vi "VM Monitor.vi"() -> ()   [LabVIEW 2022 SP3]
uses:
  <vilib>/Utility/sysdir.llb/System Directory Type.ctl
  <instrlib>/tio-labview/TIO Library/TIO Stream Open.vi
  <instrlib>/tio-labview/TIO Library/TIO RPC Send REQuest.vi
  <instrlib>/tio-labview/Labview Signal Processing/Log Binning.vi
  <instrlib>/tio-labview/TIO Library/TIO RPC Notification.vi
  <vilib>/Utility/error.llb/Clear Errors.vi
  <instrlib>/tio-labview/TIO Library/TIO RPC Parse Reply.vi
  <instrlib>/tio-labview/TIO Library/TIO RPC Parse Reply Error.vi
  <instrlib>/tio-labview/TIO Library/TIO Data Stream Parse timebase Info.vi
  <instrlib>/tio-labview/TIO Library/TIO Data Stream Parse pstream Info.vi
  <instrlib>/tio-labview/TIO Library/TIO Data Stream Parse dstream Info.vi
  <vilib>/Utility/High Resolution Relative Seconds.vi
  <instrlib>/tio-labview/TIO Library/TIO Serial Port Name Search.vi
  <instrlib>/tio-labview/TIO Library/TIO Stream Write.vi
  <instrlib>/tio-labview/TIO Library/TIO RPC Form Request.vi
  <instrlib>/tio-labview/Labview Signal Processing/Log Range.vi
  <instrlib>/tio-labview/TIO Library/TIO SLIP Serial Write.vi
  <instrlib>/tio-labview/TIO Library/TIO Form Packet.vi
  <instrlib>/tio-labview/TIO Library/TIO SLIP Encode.vi
  <instrlib>/tio-labview/TIO Library/TIO Serial Checksum CRC32.vi
  <vilib>/Utility/tcp.llb/UDP Multicast Open.vi
  <vilib>/Utility/tcp.llb/UDP Multicast Read-Write Open.vi
  <instrlib>/tio-labview/TIO Library/TIO Serial Port Discovery.vi
  <vilib>/Instr/_visa.llb/VISA Configure Serial Port (Instr).vi
  <instrlib>/tio-labview/TIO Library/TIO RPC Blocking.vi
  <vilib>/Analysis/6fits.llb/General Polynomial Fit.vi
  <vilib>/measure/maspectr.llb/FFT Power Spectrum and PSD.vi
  <vilib>/measure/maspectr.llb/FFT Power Spectrum and PSD for 1 Chan.vi
  <instrlib>/tio-labview/TIO Library/TIO Stream Read Non-blocking.vi
  <instrlib>/tio-labview/TIO Library/TIO RPC Send Heartbeat.vi
panel:
  in  "Data Rate":dbl[unit]=1000.0
  in  "Reset":bool
  in  "Log":bool
  in  "Log to file":path
  in  "URL":refnum<visa-resource-name>="tcp://localhost"
  in  "Quit":bool
  in  "Duration":dbl[unit]=1000.0
  out "T":dbl[unit]=35.88999938964844 format="%_4g"
  out "gz":dbl[unit]=-0.004659709835278764 format="%_4p"
  out "gy":dbl[unit]=-0.022590839449213182 format="%_4p"
  out "gx":dbl[unit]=-0.019901542485926807 format="%_4p"
  out "az":dbl[unit]=0.00052925927734375 format="%_4g"
  out "ay":dbl[unit]=-0.00082588623046875 format="%_4g"
  out "ax":dbl[unit]=9.998315429687501e-05 format="%_4g"
  out "P":dbl[unit]=106140.01245117188 format="%_6g"
  out "BX":dbl[unit]=3.6740006401538853e-09 format="%_6g"
  out "BY":dbl[unit]=-5.247936037597656e-07 format="%_6g"
  out "BZ":dbl[unit]=-4.973549954223633e-07 format="%_6g"
  out "B":dbl[unit]=7.230379266504588e-07 format="%_6g"
  out "Field X":T1(graph)
  out "Field Y":T1(graph)
  out "Field Z":T1(graph)
  out "Field Total":T1(graph)
  out "ID":string="Twinleaf VM4 R4"
  in  "Bin":bool=TRUE
  out "XY Graph":T2(graph)
  # "VM Monitor"
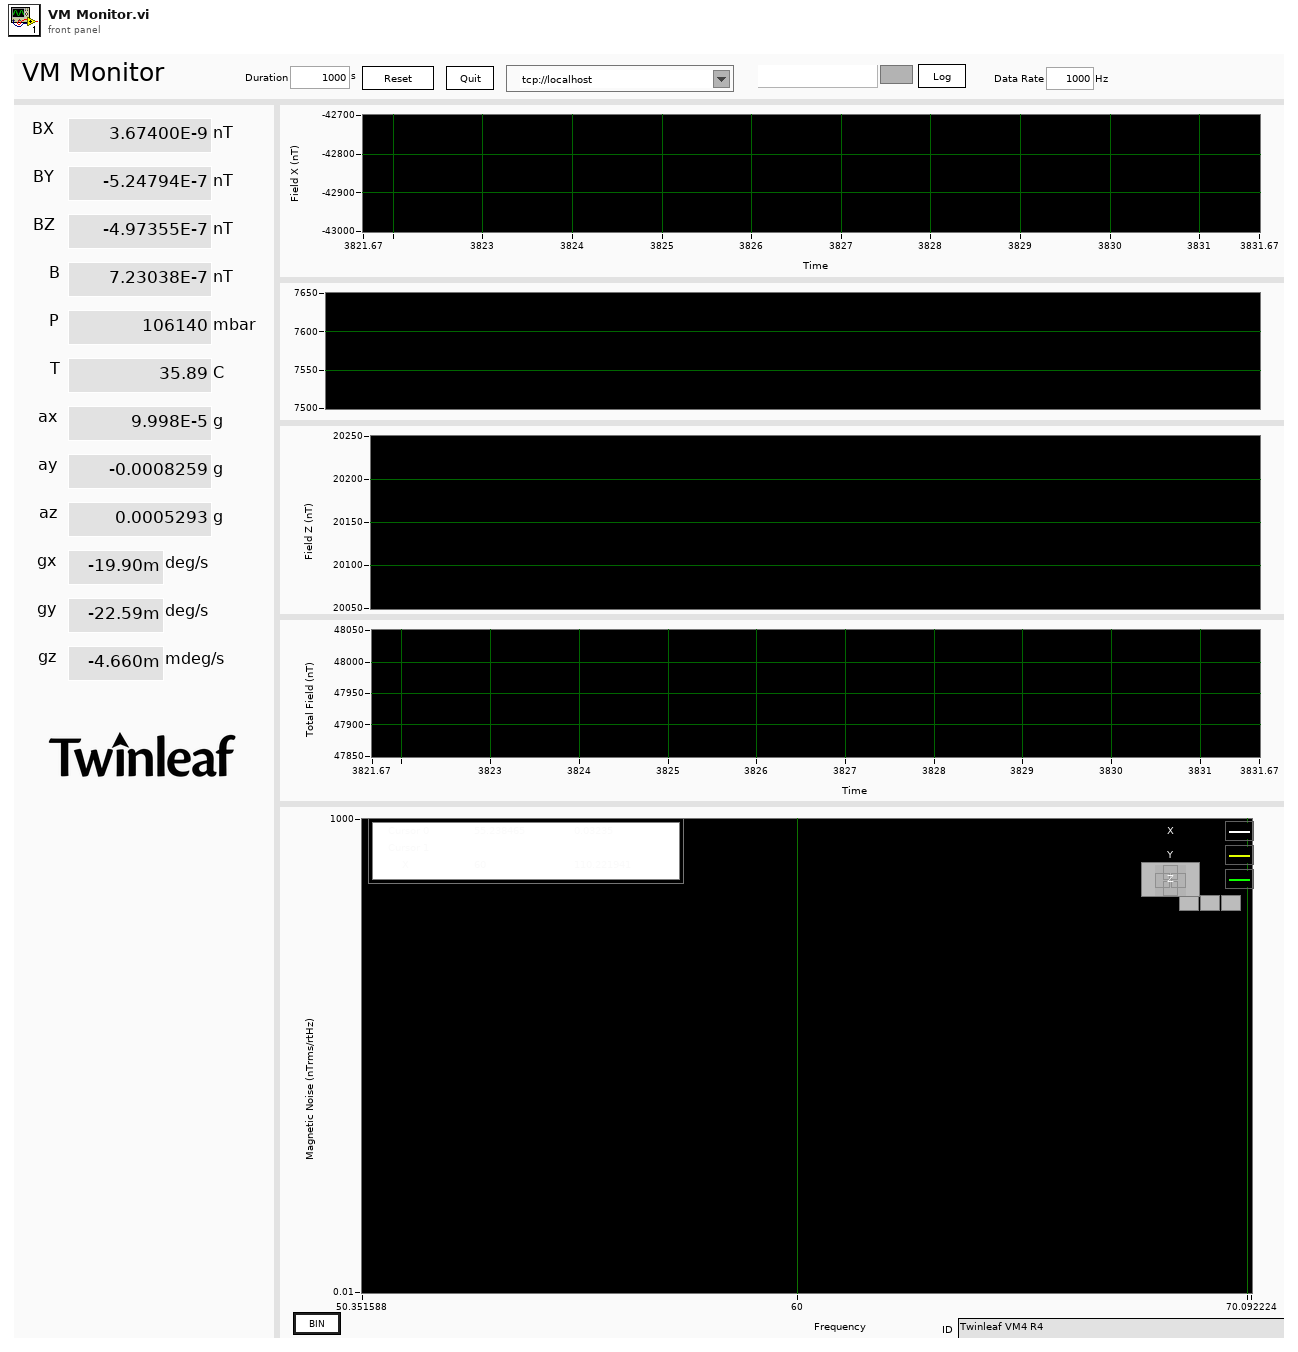
[diagram p1: front panel]
types:
  T1 = cluster{"start":dbl, "dt":dbl, "Timeseries":dbl[]}
  T2 = cluster{"Frequencies Binned":dbl[], "Spectrum Binned":dbl[]}[]
  T3 = cluster{"Awaiting REP":bool, "REQ ID":u32, "streams in":cluster{"id":u16, "timebase id":u16, "period":u32, "offset":u32, "sample number":u64, "total components":u16, "flags":u16, "components":cluster{"source id":u16, "flags":u16, "period":u32, "offset":u32}[]}[], "sources":cluster{"id":u16, "timebase_id":u16, "period":u32, "offset":u32, "fmt":i32, "flags":u16, "channels":u16, "type":u8, "name":string, "column names":string[], "title":string, "units":string}[], "timebases":cluster{"id":u16, "source":u8, "epoch":u8, "start time":u64, "period numerator (µs)":u32, "period denominator (µs)":u32, "flags":u32, "stability":sgl, "source id":string}[]}
  T4 = typedef "System Directory Type.ctl" = i32
  T5 = cluster{"TS Connection":cluster{"Type":enum16{"Serial", "TCP", "UDP", "mUDP"}, "URL":refnum<visa-resource-name>, "TO":u32, "Addr":u32, "Port":i32, "TCP":refnum<k5>, "UDP":refnum<k16>, "Route":string}, "REQ":refnum<queue>, "REP":refnum<queue>}
  T6 = cluster{"start":dbl, "dt":dbl, "Timeseries":sgl[][]}
  T7 = cluster{"stream ID":u16, "Sample Number":u32, "Raw Data":string}
  T8 = cluster{"TC Connection":cluster{"Type":enum16{"Serial", "TCP", "UDP", "mUDP"}, "URL":refnum<visa-resource-name>, "TO":u32, "Addr":u32, "Port":i32, "TCP":refnum<k5>, "UDP":refnum<k16>, "Route":string}, "REQ":refnum<queue>, "REP":refnum<queue>}
  T9 = cluster{"Name":string, "Waveform":cluster{"start":dbl, "dt":dbl, "Timeseries":dbl[][]}}[]
  T10 = cluster{"start":dbl, "dt":dbl, "Timeseries":dbl[][]}
  T11 = cluster{"Frequencies Binned":dbl[], "Spectrum Binned":dbl[]}
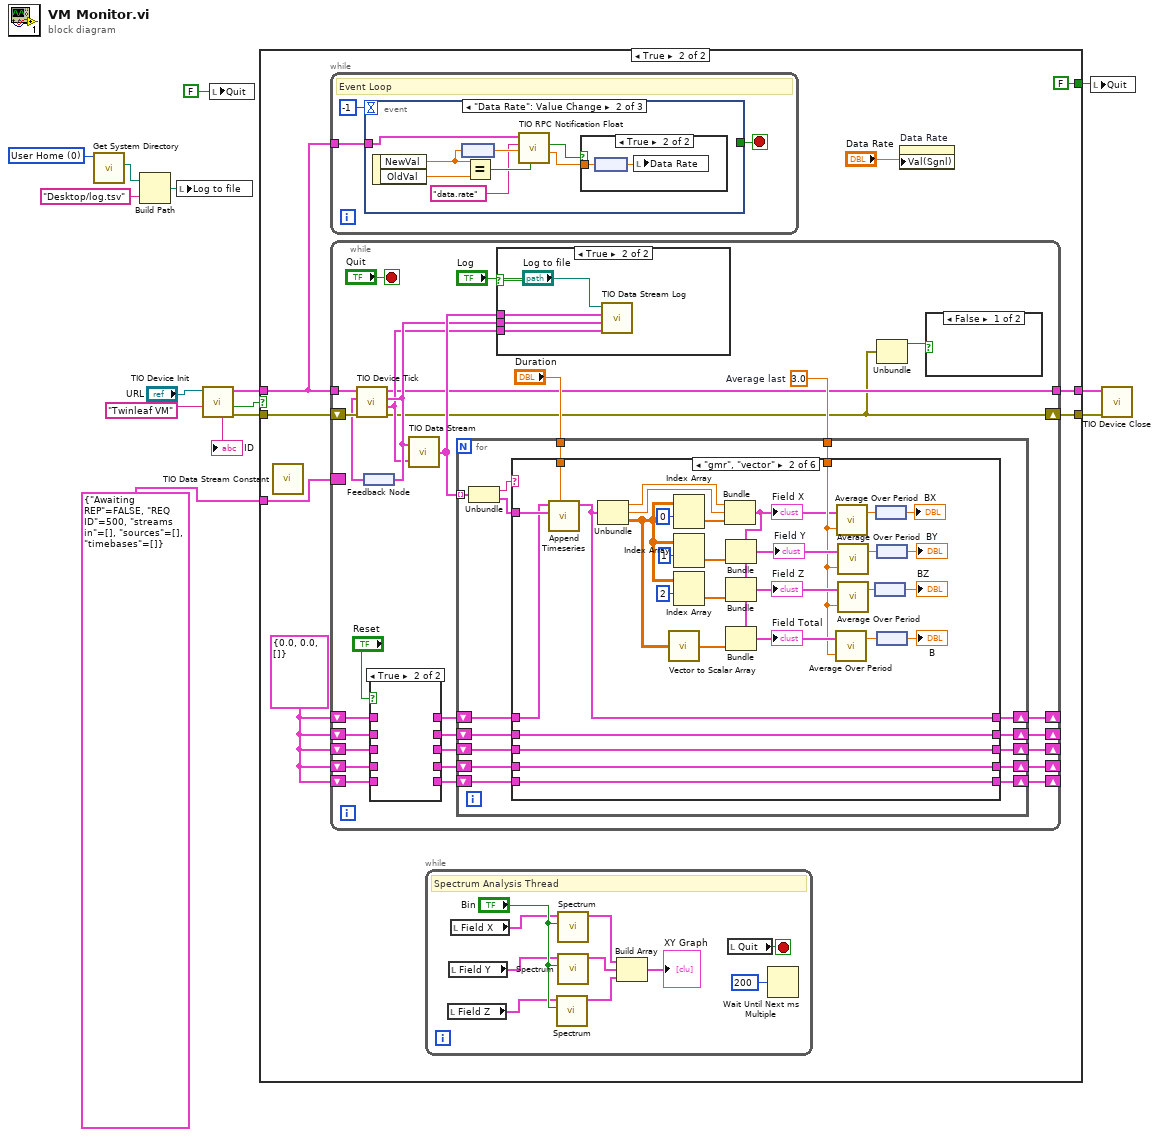
[diagram p0: block diagram]
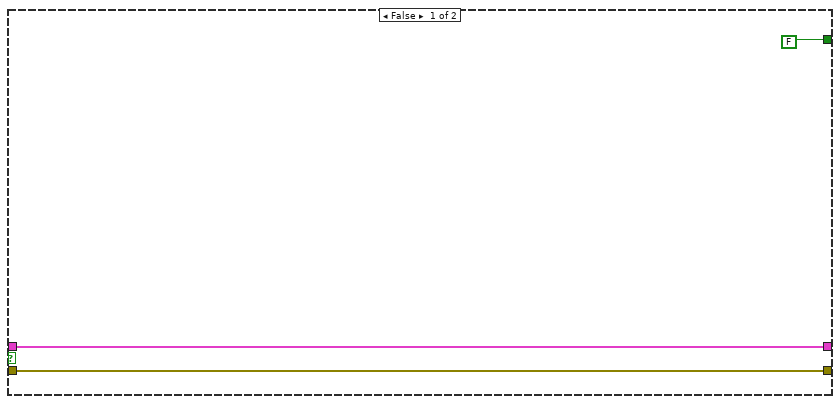
[diagram p2: hidden frame]
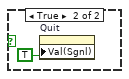
[diagram p3: hidden frame]
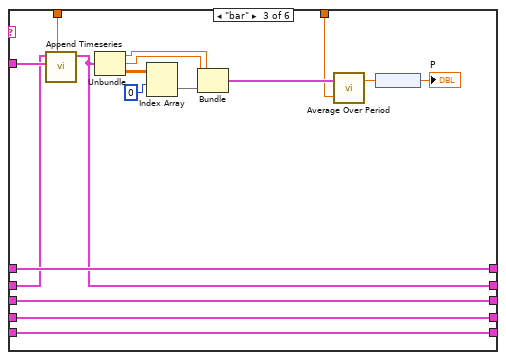
[diagram p6: hidden frame]
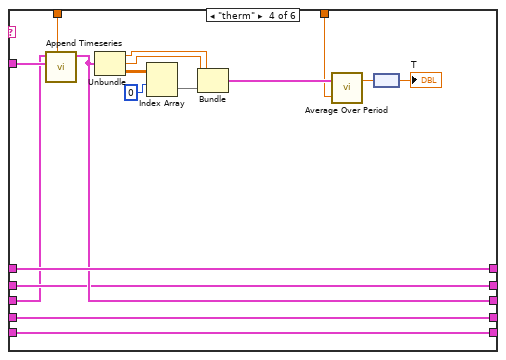
[diagram p7: hidden frame]
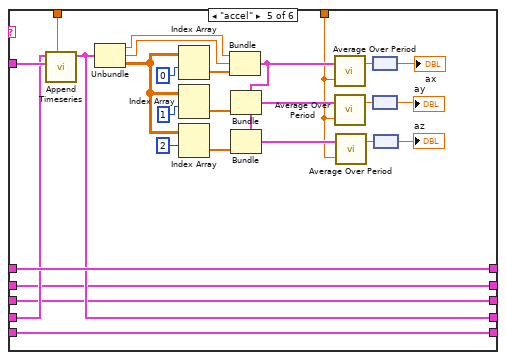
[diagram p8: hidden frame]
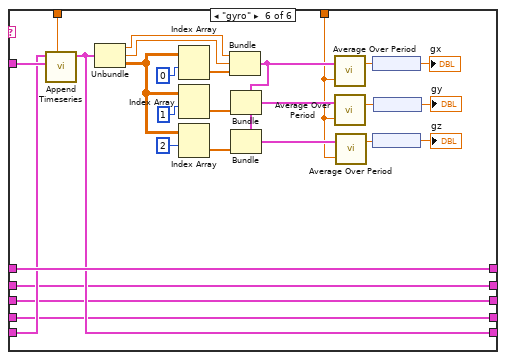
[diagram p9: hidden frame]
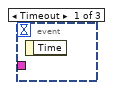
[diagram p11: hidden frame]
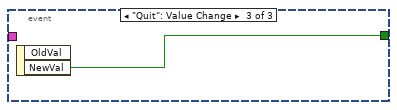
[diagram p13: hidden frame]
diagram:
  w9 = T4 0 items=["User Home"=0, "User Desktop"=1, "User Documents"=2, "User Application Data"=3, "User Preferences"=4, "User Temporary"=5, "Public Documents"=6, "Public Application Data"=7, "Public Preferences"=8, "Public Cache"=13, "System Core Libraries"=9, "System Installed Libraries"=10, "Application Files"=11, "Boot Volume Root"=12] ("system directory type")
  n1 = call <vilib>:"Get System Directory.vi"("system directory type"=w9) -> ("system directory"=w8:path)  [unwired: 10 in]
  n2 = Build Path(base path=w8, name or relative path="Desktop/log.tsv") -> (appended path=w6:path)
  n3 = local write "Log to file"(w6) -> ()
  n4 = call <instrlib>:"TIO Device Init.vi"("ID"="Twinleaf VM" ("Prefix"), "URL"="URL") -> ("error out"=w14:errorcluster, "Connected"=w2:bool, "TIO"=w15:T5, "ID Verified"=→"ID":string)  [unwired: 5 in, 1 out]
  n5 = local write "Quit"(FALSE ("Kill")) -> ()
  n6 = case shown="True" w2 {
    tunnel: w15 -> [w17 w25]
    tunnel: w14 -> [w16 w26]
    tunnel: [FALSE FALSE ("Kill")] -> w10
    tunnel: [w17 w22] -> w4
    tunnel: [w16 w21] -> w5
    tunnel: T3 {"Awaiting REP"=FALSE, "REQ ID"=500, "streams in"=[], "sources"=[], "timebases"=[]} ("TIO State") -> [_ w20]
    frame False {
    }
    frame True {
      w23 = T6 {"start"=0.0, "dt"=0.0, "Timeseries"=[]}
      n7 = call <instrlib>:"TIO Data Stream Constant.vi"() -> ()  [unwired: 1 out]
      n8 = while {
        tunnel: w25 -> [w206]
        stop <- w205 stop-if-true
        # "Event Loop"
        n9 = event shown="[1] \"Data Rate\": Value Change" {
          selector: _ -> [_ _ _]
          dyn-events: _ -> [_ _ _]
          timeout: -1 -> [_ _ _]
          tunnel: w206 -> [_ w210 _]
          tunnel: [_ _ w218] -> w205
          event Timeout {
            n10 = event-data() -> ()  [unwired: 1 in, 1 out]
          }
          event "Data Rate": Value Change {
            n11 = event-data() -> ("NewVal"=w212:dbl[unit], "OldVal"=w214:dbl[unit])  [unwired: 1 in]
            n12 = node(w212) -> (w211:dbl)
            n13 = Equal?(x=w212, y=w214) -> (x = y?=w215:bool)
            n14 = call <instrlib>:"TIO RPC Notification Float.vi"("Read"=w215, "Set value"=w211, "Topic"="data.rate", "TIO"=w210) -> ("Get value (default if error)"=w213:sgl, "Response"=w208:bool)  [unwired: 4 in, 1 out]
            n15 = case shown="True" w208 {
              tunnel: w213 -> [_ w217]
              frame False {
              }
              frame True {
                n16 = node(w217) -> (w216:sgl[unit])
                n17 = local write "Data Rate"(w216) -> ()
              }
            }
          }
          event "Quit": Value Change {
            n18 = event-data() -> ("NewVal"=w218:bool)  [unwired: 1 in, 1 out]
          }
        }
      }
      n19 = while {
        tunnel: w25 -> [w55]
        shift-right: [w51] -> _
        shift-left: w23 -> [w39]
        shift-right: [w48] -> _
        shift-left: w23 -> [w38]
        shift-right: [w47] -> _
        shift-left: w23 -> [w37]
        shift-right: [w46] -> _
        shift-left: w23 -> [w36]
        shift-right: [w45] -> _
        shift-left: w23 -> [w35]
        border: w20 -> [_]
        tunnel: [w29] -> w22
        shift-right: [w28] -> w21
        shift-left: w26 -> [w54]
        stop <- "Quit" stop-if-true
        w50 = dbl[unit] 3.0  # Average last
        n20 = feedback #1() -> (w44:T3)
        n21 = call <instrlib>:"TIO Device Tick.vi"("Error in"=w54, "TIO State"=w44, "TIO"=w55) -> ("Error out"=w28:errorcluster, "Data Out"=w41:T7, "TIO State"=w42:T3, "TIO"=w29:T8)  [unwired: 5 in]
        n22 = feedback-in #1(w42) -> ()
        n23 = case shown="True" "Reset" {
          tunnel: w39 -> [w61 _]
          tunnel: w38 -> [w60 _]
          tunnel: w37 -> [w59 _]
          tunnel: w36 -> [w58 _]
          tunnel: w35 -> [w57 _]
          tunnel: [w57 _] -> w34
          tunnel: [w58 _] -> w33
          tunnel: [w59 _] -> w32
          tunnel: [w60 _] -> w31
          tunnel: [w61 _] -> w30
          frame False {
          }
          frame True {
          }
        }
        n24 = call <instrlib>:"TIO Data Stream.vi"("Raw Data"=w41, "TIO State"=w42) -> ("Data Out"=w43:T9)
        n25 = for {
          tunnel: "Duration" -> [w76]
          tunnel: w50 -> [w73]
          tunnel: w43 -> [w64] mode=indexing
          shift-right: [w75] -> w51
          shift-left: w30 -> [w74]
          shift-right: [w72] -> w48
          shift-left: w31 -> [w71]
          shift-right: [w70] -> w47
          shift-left: w32 -> [w69]
          shift-right: [w68] -> w46
          shift-left: w33 -> [w67]
          shift-right: [w66] -> w45
          shift-left: w34 -> [w65]
          n26 = Unbundle(w64) -> ("Name"=w63:string, "Waveform"=w62:T10)
          n27 = case shown="\"gmr\", \"vector\"" w63 {
            tunnel: w76 -> [_ w112 w129 w146 w173 w200]
            tunnel: w73 -> [_ w93 w118 w136 w152 w185]
            tunnel: w62 -> [_ w88 w122 w140 w156 w189]
            tunnel: [w81 w87 w121 w139 w153 w186] -> w75
            tunnel: w74 -> [w81 w86 w121 w139 w153 w186]
            tunnel: [w80 w85 w117 w133 w149 w176] -> w72
            tunnel: w71 -> [w80 w85 w116 w133 w149 w176]
            tunnel: [w79 w84 w115 w134 w148 w175] -> w70
            tunnel: w69 -> [w79 w84 w115 w132 w148 w175]
            tunnel: [w78 w83 w114 w131 w151 w174] -> w68
            tunnel: w67 -> [w78 w83 w114 w131 w150 w174]
            tunnel: [w77 w82 w113 w130 w147 w178] -> w66
            tunnel: w65 -> [w77 w82 w113 w130 w147 w177]
            frame Default {
            }
            frame "gmr", "vector" {
              n28 = call <instrlib>:"Append Timeseries.vi"("Duration"=w112, "In New"=w88, "In Old"=w86) -> ("Appended"=w87:T10)  [unwired: 8 in]
              n29 = Unbundle(w87) -> ("start"=w111:dbl, "dt"=w92:dbl, "Timeseries"=w90:dbl[][])
              n30 = call <instrlib>:"Vector to Scalar Array.vi"("Three axis vector"=w90) -> ("Total field"=w89:dbl[])
              n31 = Index Array(array=w90, index (row)=0 ("disabled index (col)")) -> (element=w107:dbl[])  [unwired: 1 in]
              n32 = Index Array(array=w90, index (row)=1 ("disabled index (col)")) -> (element=w106:dbl[])  [unwired: 1 in]
              n33 = Index Array(array=w90, index (row)=2 ("disabled index (col)")) -> (element=w105:dbl[])  [unwired: 1 in]
              n34 = Bundle("start"=w111, "dt"=w92, "Timeseries"=w107) -> (w91:T1)  [unwired: 1 in]
              "Field X" <- w91
              n35 = Bundle(cluster=w91, "Timeseries"=w106) -> (w102:T1)  [unwired: 2 in]
              "Field Y" <- w102
              n36 = Bundle(cluster=w91, "Timeseries"=w105) -> (w101:T1)  [unwired: 2 in]
              "Field Z" <- w101
              n37 = Bundle(cluster=w91, "Timeseries"=w89) -> (w100:T1)  [unwired: 2 in]
              "Field Total" <- w100
              n38 = call <instrlib>:"Average Over Period.vi"("Average Period"=w93, "Waveform"=w100) -> ("Average"=w95:dbl)  [unwired: 1 in]
              n39 = call <instrlib>:"Average Over Period.vi"("Average Period"=w93, "Waveform"=w91) -> ("Average"=w104:dbl)  [unwired: 1 in]
              n40 = call <instrlib>:"Average Over Period.vi"("Average Period"=w93, "Waveform"=w102) -> ("Average"=w99:dbl)  [unwired: 1 in]
              n41 = call <instrlib>:"Average Over Period.vi"("Average Period"=w93, "Waveform"=w101) -> ("Average"=w97:dbl)  [unwired: 1 in]
              n42 = node(w97) -> (→"BZ":dbl[unit])
              n43 = node(w104) -> (→"BX":dbl[unit])
              n44 = node(w99) -> (→"BY":dbl[unit])
              n45 = node(w95) -> (→"B":dbl[unit])
            }
            frame "bar" {
              n46 = call <instrlib>:"Append Timeseries.vi"("Duration"=w129, "In New"=w122, "In Old"=w116) -> ("Appended"=w117:T10)  [unwired: 8 in]
              n47 = Unbundle(w117) -> ("start"=w127:dbl, "dt"=w128:dbl, "Timeseries"=w120:dbl[][])
              n48 = Index Array(array=w120, index (row)=0 ("disabled index (col)")) -> (element=w125:dbl[])  [unwired: 1 in]
              n49 = Bundle("start"=w127, "dt"=w128, "Timeseries"=w125) -> (w119:T1)  [unwired: 1 in]
              n50 = call <instrlib>:"Average Over Period.vi"("Average Period"=w118, "Waveform"=w119) -> ("Average"=w123:dbl)  [unwired: 1 in]
              n51 = node(w123) -> (→"P":dbl[unit])
            }
            frame "therm" {
              n52 = call <instrlib>:"Append Timeseries.vi"("Duration"=w146, "In New"=w140, "In Old"=w132) -> ("Appended"=w134:T10)  [unwired: 8 in]
              n53 = Unbundle(w134) -> ("start"=w144:dbl, "dt"=w145:dbl, "Timeseries"=w138:dbl[][])
              n54 = Index Array(array=w138, index (row)=0 ("disabled index (col)")) -> (element=w142:dbl[])  [unwired: 1 in]
              n55 = Bundle("start"=w144, "dt"=w145, "Timeseries"=w142) -> (w137:T1)  [unwired: 1 in]
              n56 = call <instrlib>:"Average Over Period.vi"("Average Period"=w136, "Waveform"=w137) -> ("Average"=w141:dbl)  [unwired: 1 in]
              n57 = node(w141) -> (→"T":dbl[unit])
            }
            frame "accel" {
              n58 = call <instrlib>:"Append Timeseries.vi"("Duration"=w173, "In New"=w156, "In Old"=w150) -> ("Appended"=w151:T10)  [unwired: 8 in]
              n59 = Unbundle(w151) -> ("start"=w171:dbl, "dt"=w172:dbl, "Timeseries"=w155:dbl[][])
              n60 = Index Array(array=w155, index (row)=0 ("disabled index (col)")) -> (element=w168:dbl[])  [unwired: 1 in]
              n61 = Index Array(array=w155, index (row)=1 ("disabled index (col)")) -> (element=w167:dbl[])  [unwired: 1 in]
              n62 = Index Array(array=w155, index (row)=2 ("disabled index (col)")) -> (element=w164:dbl[])  [unwired: 1 in]
              n63 = Bundle("start"=w171, "dt"=w172, "Timeseries"=w168) -> (w154:T1)  [unwired: 1 in]
              n64 = Bundle(cluster=w154, "Timeseries"=w167) -> (w165:T1)  [unwired: 2 in]
              n65 = Bundle(cluster=w154, "Timeseries"=w164) -> (w162:T1)  [unwired: 2 in]
              n66 = call <instrlib>:"Average Over Period.vi"("Average Period"=w152, "Waveform"=w154) -> ("Average"=w163:dbl)  [unwired: 1 in]
              n67 = call <instrlib>:"Average Over Period.vi"("Average Period"=w152, "Waveform"=w165) -> ("Average"=w160:dbl)  [unwired: 1 in]
              n68 = call <instrlib>:"Average Over Period.vi"("Average Period"=w152, "Waveform"=w162) -> ("Average"=w159:dbl)  [unwired: 1 in]
              n69 = node(w163) -> (→"ax":dbl[unit])
              n70 = node(w160) -> (→"ay":dbl[unit])
              n71 = node(w159) -> (→"az":dbl[unit])
            }
            frame "gyro" {
              n72 = call <instrlib>:"Append Timeseries.vi"("Duration"=w200, "In New"=w189, "In Old"=w177) -> ("Appended"=w178:T10)  [unwired: 8 in]
              n73 = Unbundle(w178) -> ("start"=w198:dbl, "dt"=w199:dbl, "Timeseries"=w188:dbl[][])
              n74 = Index Array(array=w188, index (row)=0 ("disabled index (col)")) -> (element=w195:dbl[])  [unwired: 1 in]
              n75 = Index Array(array=w188, index (row)=1 ("disabled index (col)")) -> (element=w194:dbl[])  [unwired: 1 in]
              n76 = Index Array(array=w188, index (row)=2 ("disabled index (col)")) -> (element=w191:dbl[])  [unwired: 1 in]
              n77 = Bundle("start"=w198, "dt"=w199, "Timeseries"=w195) -> (w187:T1)  [unwired: 1 in]
              n78 = Bundle(cluster=w187, "Timeseries"=w194) -> (w192:T1)  [unwired: 2 in]
              n79 = Bundle(cluster=w187, "Timeseries"=w191) -> (w190:T1)  [unwired: 2 in]
              n80 = call <instrlib>:"Average Over Period.vi"("Average Period"=w185, "Waveform"=w187) -> ("Average"=w181:dbl)  [unwired: 1 in]
              n81 = call <instrlib>:"Average Over Period.vi"("Average Period"=w185, "Waveform"=w192) -> ("Average"=w180:dbl)  [unwired: 1 in]
              n82 = call <instrlib>:"Average Over Period.vi"("Average Period"=w185, "Waveform"=w190) -> ("Average"=w179:dbl)  [unwired: 1 in]
              n83 = node(w181) -> (→"gx":dbl[unit])
              n84 = node(w179) -> (→"gz":dbl[unit])
              n85 = node(w180) -> (→"gy":dbl[unit])
            }
          }
        }
        n86 = case shown="True" "Log" {
          tunnel: w43 -> [_ w202]
          tunnel: w42 -> [_ w203]
          tunnel: w41 -> [_ w201]
          frame False {
          }
          frame True {
            n87 = call <instrlib>:"TIO Data Stream Log.vi"(8:"Data Out"=w201, "TIO State"=w203, 10:"Data Out"=w202, "Log to file"="Log to file") -> ()  [unwired: 8 in]
          }
        }
        n88 = Unbundle(w28) -> ("status"=w27:bool)  [unwired: 2 out]
        n89 = case shown="False" w27 {
          frame False {
          }
          frame True {
            n90 = property on="Quit" class="Bool (strict)"("Val(Sgnl)"=TRUE ("Value (Signaling)")) -> ()  [unwired: 2 in, 2 out]
          }
        }
      }
      n91 = while {
        stop <- w222 stop-if-true
        # "Spectrum Analysis Thread"
        n92 = local read "Field Z"() -> (w219:T1)
        n93 = local read "Field Y"() -> (w220:T1)
        n94 = local read "Field X"() -> (w221:T1)
        n95 = call <instrlib>:"Spectrum.vi"("Binning"="Bin", "Waveform 1"=w219) -> ("Cluster"=w224:T11)  [unwired: 7 in]
        n96 = call <instrlib>:"Spectrum.vi"("Binning"="Bin", "Waveform 1"=w221) -> ("Cluster"=w226:T11)  [unwired: 7 in]
        n97 = call <instrlib>:"Spectrum.vi"("Binning"="Bin", "Waveform 1"=w220) -> ("Cluster"=w225:T11)  [unwired: 7 in]
        n98 = Build Array(w226, w225, w224) -> (→"XY Graph":T2)
        n99 = local read "Quit"() -> (w222:bool)
        n100 = Wait Until Next ms Multiple(millisecond multiple=u32 200) -> ()  [unwired: 1 out]
      }
      n101 = property on="Data Rate" class="DigNum (strict)"("Val(Sgnl)"="Data Rate") -> ()  [unwired: 2 in, 2 out]
    }
  }
  n102 = local write "Quit"(w10) -> ()
  n103 = call <instrlib>:"TIO Device Close.vi"("Error in"=w5, "TIO"=w4) -> ()  [unwired: 10 in]
